vi "Inter-Move Items.vi"(4 "indent":i32, 6 "Insertion index":i32, 7 "BetterHandle in (source)":refnum<class "BetterHandle.lvclass">, 8 "error in (no error)":errorcluster, 9 "Copy?":bool, 10 "Indices to move":i32[](array[numeric]), 11 "BetterHandle in (destination)":refnum<class "BetterHandle.lvclass">) -> (0 "error out":errorcluster, 3 "BetterHandle out (destination)":refnum<class "BetterHandle.lvclass">, 5 "BetterHandle out (source)":refnum<class "BetterHandle.lvclass">)   [LabVIEW 2020, in "BetterDragAndDrop.lvlib" / "BetterHandle.lvclass"]
uses:
  BetterHandle.lvclass
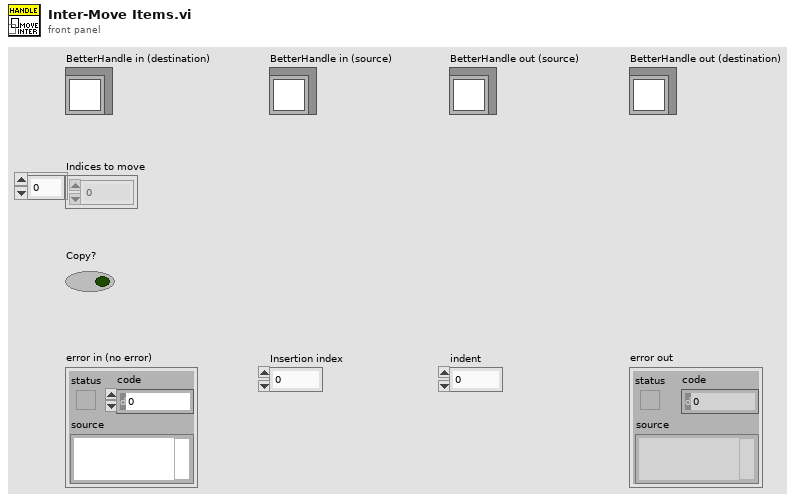
[diagram p1: front panel]
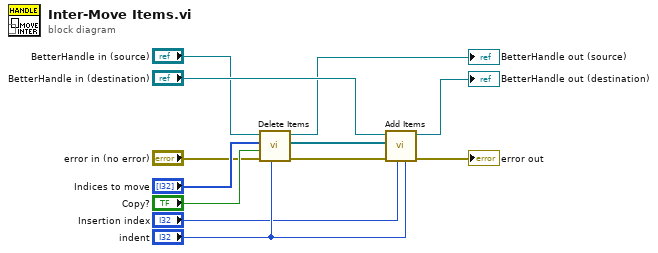
[diagram p0: block diagram]
diagram:
  n1 = call-dynamic "Delete Items.vi"("indent"="indent", "error in (no error)"="error in (no error)", "Copy? (F)"="Copy?", "Indices to remove"="Indices to move", "BetterHandle in"="BetterHandle in (source)") -> ("error out"=w7:errorcluster, "items removed"=w10:refnum<class "BetterItem.lvclass">[], "BetterHandle out"=→"BetterHandle out (source)":refnum<class "BetterHandle.lvclass">)  [unwired: 4 in]
  n2 = call-dynamic "Add Items.vi"("indent"="indent", "Insertion index"="Insertion index", "error in (no error)"=w7, "Items to Add"=w10, "BetterHandle in"="BetterHandle in (destination)") -> ("error out"=→"error out":errorcluster, "BetterHandle out"=→"BetterHandle out (destination)":refnum<class "BetterHandle.lvclass">)  [unwired: 5 in]
